vi "Config Write Sequence Steps.vi"() -> ()   [LabVIEW 2012]
uses:
  <vilib>/Utility/config.llb/Write Key (String).vi
  <vilib>/Utility/config.llb/NI_LVConfig.lvlib
panel:
  in  "Error In":errorcluster
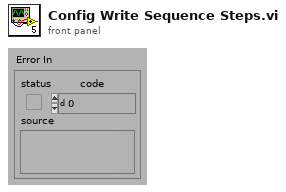
[diagram p1: front panel]
types:
  T1 = typedef "NI_LVConfig.lvlib/Config Data RefNum.ctl" = refnum<k1>
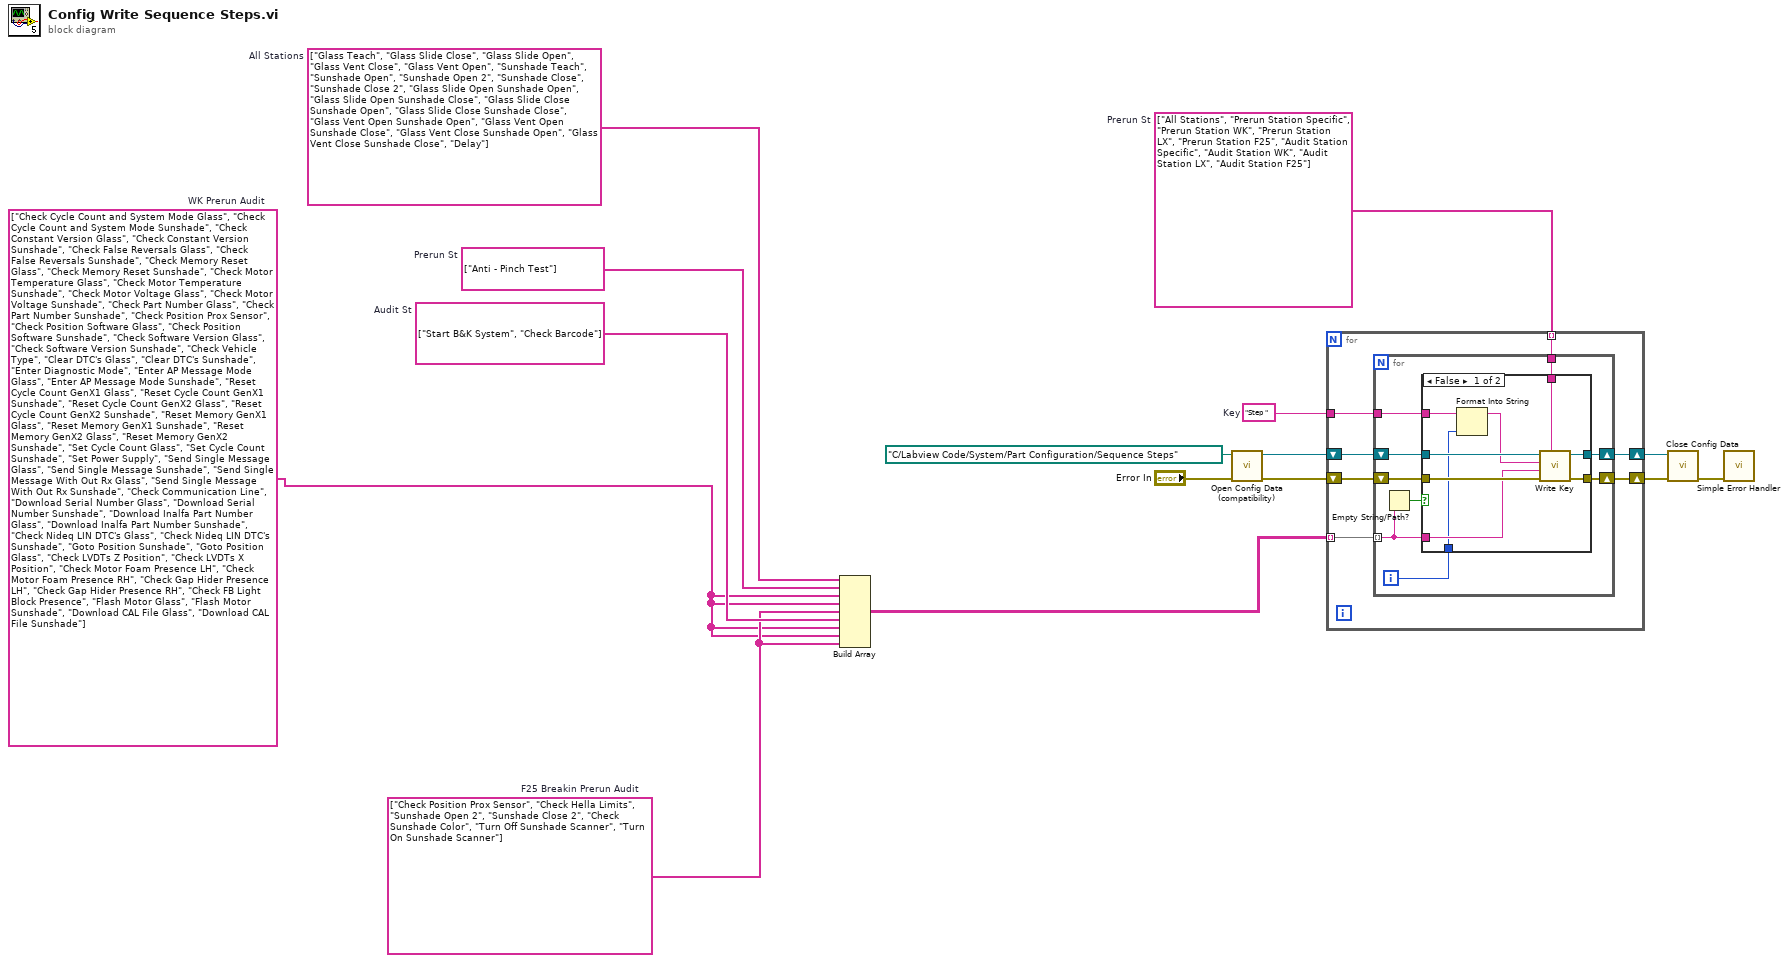
[diagram p0: block diagram]
diagram:
  w2 = string[] ["Check Position Prox Sensor", "Check Hella Limits", "Sunshade Open 2", "Sunshade Close 2", "Check Sunshade Color", "Turn Off Sunshade Scanner", "Turn On Sunshade Scanner"]  # F25 Breakin Prerun Audit
  w1 = string[] ["Check Cycle Count and System Mode Glass", "Check Cycle Count and System Mode Sunshade", "Check Constant Version Glass", "Check Constant Version Sunshade", "Check False Reversals Glass", "Check False Reversals Sunshade", "Check Memory Reset Glass", "Check Memory Reset Sunshade", "Check Motor Temperature Glass", "Check Motor Temperature Sunshade", "Check Motor Voltage Glass", "Check Motor Voltage Sunshade", "Check Part Number Glass", "Check Part Number Sunshade", "Check Position Prox Sensor", "Check Position Software Glass", "Check Position Software Sunshade", "Check Software Version Glass", "Check Software Version Sunshade", "Check Vehicle Type", "Clear DTC's Glass", "Clear DTC's Sunshade", "Enter Diagnostic Mode", "Enter AP Message Mode Glass", "Enter AP Message Mode Sunshade", "Reset Cycle Count GenX1 Glass", "Reset Cycle Count GenX1 Sunshade", "Reset Cycle Count GenX2 Glass", "Reset Cycle Count GenX2 Sunshade", "Reset Memory GenX1 Glass", "Reset Memory GenX1 Sunshade", "Reset Memory GenX2 Glass", "Reset Memory GenX2 Sunshade", "Set Cycle Count Glass", "Set Cycle Count Sunshade", "Set Power Supply", "Send Single Message Glass", "Send Single Message Sunshade", "Send Single Message With Out Rx Glass", "Send Single Message With Out Rx Sunshade", "Check Communication Line", "Download Serial Number Glass", "Download Serial Number Sunshade", "Download Inalfa Part Number Glass", "Download Inalfa Part Number Sunshade", "Check Nideq LIN DTC's Glass", "Check Nideq LIN DTC's Sunshade", "Goto Position Sunshade", "Goto Position Glass", "Check LVDTs Z Position", "Check LVDTs X Position", "Check Motor Foam Presence LH", "Check Motor Foam Presence RH", "Check Gap Hider Presence LH", "Check Gap Hider Presence RH", "Check FB Light Block Presence", "Flash Motor Glass", "Flash Motor Sunshade", "Download CAL File Glass", "Download CAL File Sunshade"]  # WK Prerun Audit
  w3 = string[] ["Glass Teach", "Glass Slide Close", "Glass Slide Open", "Glass Vent Close", "Glass Vent Open", "Sunshade Teach", "Sunshade Open", "Sunshade Open 2", "Sunshade Close", "Sunshade Close 2", "Glass Slide Open Sunshade Open", "Glass Slide Open Sunshade Close", "Glass Slide Close Sunshade Open", "Glass Slide Close Sunshade Close", "Glass Vent Open Sunshade Open", "Glass Vent Open Sunshade Close", "Glass Vent Close Sunshade Open", "Glass Vent Close Sunshade Close", "Delay"]  # All Stations
  w4 = string[] ["All Stations", "Prerun Station Specific", "Prerun Station WK", "Prerun Station LX", "Prerun Station F25", "Audit Station Specific", "Audit Station WK", "Audit Station LX", "Audit Station F25"]  # Prerun St
  w15 = "Step "  # Key
  w6 = string[] ["Start B&K System", "Check Barcode"]  # Audit St
  w7 = string[] ["Anti - Pinch Test"]  # Prerun St
  n1 = Build Array(w3, w7, w1, w1, w2, w6, w1, w1, w2) -> (w5:string[][])
  n2 = call <vilib>:"Open Config Data (compatibility).vi"("error in (no error)"="Error In", "configuration file path"=path "C:/Labview Code/System/Part Configuration/Sequence Steps") -> ("error out"=w12:errorcluster, "refnum"=w13:T1)  [unwired: 7 in, 1 out]
  n3 = for {
    tunnel: w15 -> [w22]
    tunnel: w4 -> [w17] mode=indexing
    tunnel: w5 -> [w16] mode=indexing
    shift-right: [w18] -> w9
    shift-left: w12 -> [w20]
    shift-right: [w19] -> w10
    shift-left: w13 -> [w21]
    n4 = for {
      tunnel: w22 -> [w25]
      tunnel: w17 -> [w27]
      shift-right: [w29] -> w19
      shift-left: w21 -> [w31]
      shift-right: [w28] -> w18
      shift-left: w20 -> [w30]
      tunnel: w16 -> [w24] mode=indexing
      i -> [w26]
      n5 = Empty String/Path?(string/path=w24) -> (empty?=w23:bool)
      n6 = case shown="False" w23 {
        tunnel: w31 -> [w40 w42]
        tunnel: w30 -> [w39 w41]
        tunnel: [w38 w42] -> w29
        tunnel: [w37 w41] -> w28
        tunnel: w27 -> [w36 _]
        tunnel: w24 -> [w35 _]
        tunnel: w26 -> [w34 _]
        tunnel: w25 -> [w33 _]
        frame False {
          n7 = Format Into String(initial string=w33, w34) -> (resulting string=w32:string)  [unwired: 2 in, 1 out]
          n8 = call-poly <vilib>:"Write Key.vi"("section"=w36, "error in (no error)"=w39, "value"=w35, "key"=w32, "refnum"=w40) -> ("error out"=w37:errorcluster, "refnum out"=w38:T1)  [unwired: 4 in, 1 out]
        }
        frame True {
        }
      }
    }
  }
  n9 = call <vilib>:"Close Config Data.vi"("error in (no error)"=w9, "refnum"=w10) -> ("error out"=w14:errorcluster)  [unwired: 8 in, 1 out]
  n10 = call <vilib>:"Simple Error Handler.vi"("error in (no error)"=w14) -> ()  [unwired: 4 in, 5 out]
